vi "Flush Data to Log File.vi"(8 "error in (no error)":cluster{"状态":bool, "代码":i32, "源":string} caption="错误输入（无错误）", 10 "数据队列":refnum<queue>, 11 "记录配置":T1) -> (0 "error out":cluster{"状态":bool, "代码":i32, "源":string} caption="错误输出")   [LabVIEW 2015, in "DAQ.lvlib"]
doc: "将数据队列中待处理的数据写入记录文件，并从数据队列中清空。关闭TDMS文件引用。"
uses:
  DAQ.lvlib
  Support/Logging Configuration.ctl
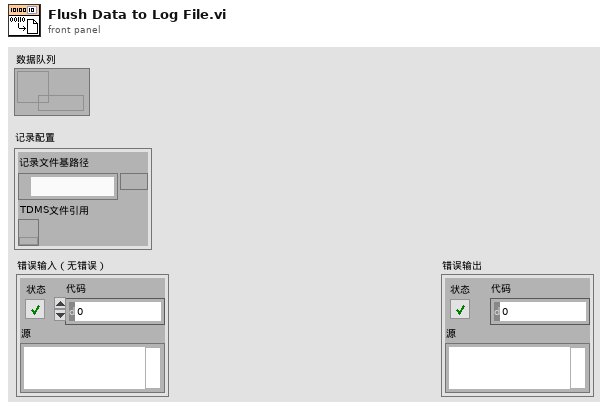
[diagram p1: front panel]
types:
  T1 = typedef "DAQ.lvlib/Logging Configuration.ctl" = cluster{"记录文件基路径":path, "TDMS文件引用":refnum<k34>}
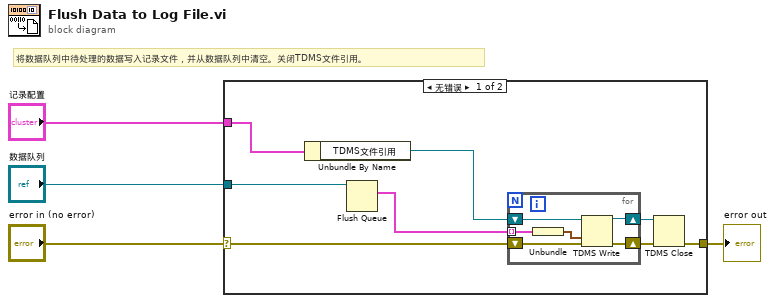
[diagram p0: block diagram]
diagram:
  # "将数据队列中待处理的数据写入记录文件，并从数据队列中清空。关闭TDMS文件引用。"
  n1 = case shown="无错误" "error in (no error)" {
    selector: "error in (no error)" -> [w5 w19]
    tunnel: "数据队列" -> [w8 _]
    tunnel: "记录配置" -> [w7 _]
    tunnel: [w6 w19] -> w2
    frame No Error {
      n2 = Unbundle By Name(w7) -> ("TDMS文件引用"=w9:refnum<k34>)
      n3 = Flush Queue(queue=w8) -> (remaining elements=w12:cluster{"Array":waveform(dbl)[]}[])  [unwired: 1 in, 2 out]
      n4 = for {
        shift-right: [w15] -> w10
        shift-left: w9 -> [w16]
        shift-right: [w17] -> w11
        shift-left: w5 -> [w18]
        tunnel: w12 -> [w14] mode=indexing
        n5 = Unbundle(w14) -> ("Array"=w13:waveform(dbl)[])
        n6 = TDMS Write(0:w16, 9:w13, 11:w18) -> (4:w15:refnum<k34>, 15:w17:errorcluster)  [unwired: 3 in, 2 out]
      }
      n7 = TDMS Close(8:w11, 11:w10) -> (0:w6:errorcluster)  [unwired: 1 out]
    }
    frame Error {
    }
  }
  "error out" <- w2
